vi "编码规则.vi"(8 "错误输入":errorcluster, 9 "编码正则表达式":string, 11 "功能":enum16{"读取", "写入"}(ring)) -> (0 "错误输出":errorcluster, 2 "正则表达式输出（多行）":string[](array[string]), 3 "正则表达式输出（单行）":string)   [LabVIEW 2020]
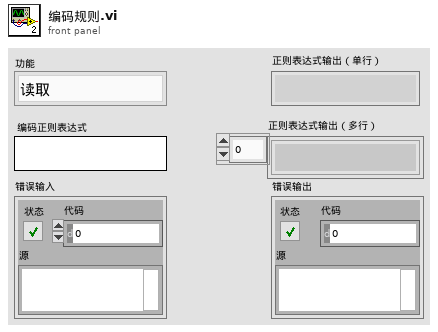
[diagram p1: front panel]
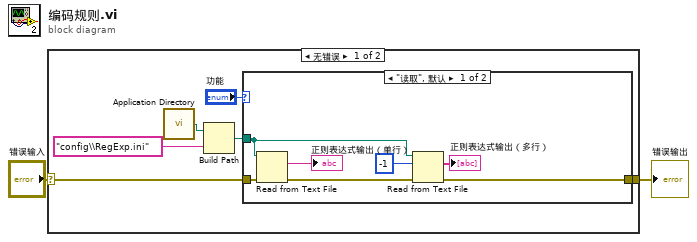
[diagram p0: block diagram]
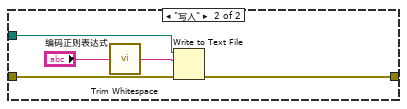
[diagram p2: hidden frame]
diagram:
  n1 = case shown="无错误" "错误输入" {
    selector: "错误输入" -> [w7 w21]
    tunnel: [w6 w21] -> w1
    frame No Error {
      n2 = call <vilib>:"Application Directory.vi"() -> ("Application Directory"=w3:path)
      n3 = Build Path(base path=w3, name or relative path="config\\RegExp.ini" ("名称或相对路径")) -> (appended path=w4:path)
      n4 = case shown="\"读取\", 默认" "功能" {
        tunnel: w4 -> [w9 w17]
        tunnel: w7 -> [w14 w19]
        tunnel: [w12 w18] -> w6
        frame "读取", Default {
          n5 = Read from Text File(file (use dialog)=w9, error in=w14) -> (text=→"正则表达式输出（单行）":string, error out=w13:errorcluster)  [unwired: 2 in, 2 out]
          n6 = Read from Text File(file (use dialog)=w9, count=-1 ("计数"), error in=w13) -> (text=→"正则表达式输出（多行）":string[], error out=w12:errorcluster)  [unwired: 1 in, 2 out]
        }
        frame "写入" {
          n7 = call <vilib>:"Trim Whitespace.vi"("string"="编码正则表达式") -> ("trimmed string"=w20:string)  [unwired: 1 in]
          n8 = Write to Text File(file (use dialog)=w17, text=w20, error in=w19) -> (error out=w18:errorcluster)  [unwired: 1 in, 2 out]
        }
      }
    }
    frame Error {
    }
  }
  "错误输出" <- w1
